vi "GetLastTotalGames.vi"(8 "error in (no error)":errorcluster, 11 "ClashRoyale in":refnum<class "ClashRoyale.lvclass">) -> (0 "error out":errorcluster, 2 "Last Total Games":i64, 3 "ClashRoyale out":refnum<class "ClashRoyale.lvclass">)   [LabVIEW 2020, in "ClashRoyale.lvclass"]
uses:
  ClashRoyale.lvclass
  <vilib>/drjdpowell/SQLite Library/SQLite.lvlib
  <vilib>/drjdpowell/SQLite Library/SQL Connection/Execute SQL (Single Integer).vi
  <vilib>/drjdpowell/SQLite Library/SQL Connection/Connection.lvclass
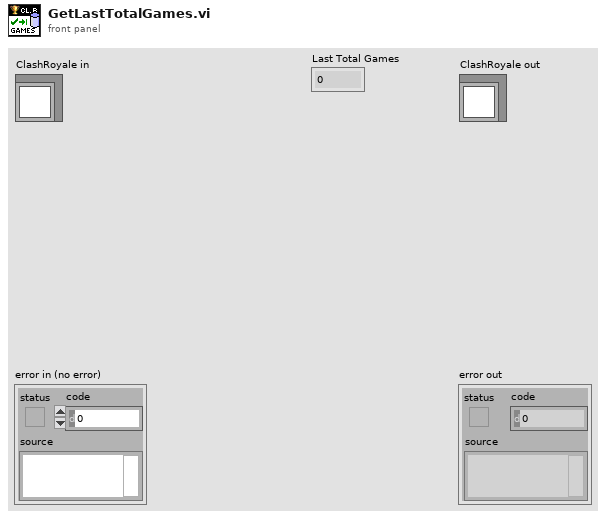
[diagram p1: front panel]
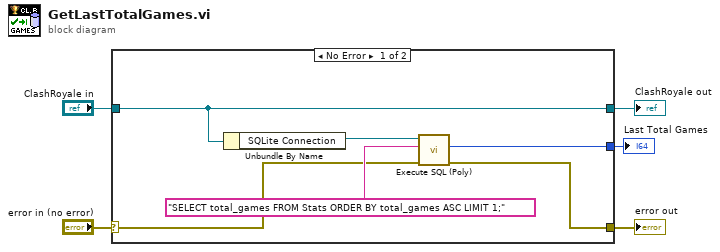
[diagram p0: block diagram]
diagram:
  n1 = case shown="No Error" "error in (no error)" {
    selector: "error in (no error)" -> [w7 w13]
    tunnel: [w6 w13] -> w4
    tunnel: [w11 w12] -> w2
    tunnel: "ClashRoyale in" -> [w11 w12]
    tunnel: [w8 _] -> w1
    frame No Error {
      n2 = Unbundle By Name(w11) -> ("SQLite Connection"=w10:refnum<class "Connection.lvclass">)
      n3 = call-poly <vilib>:"Execute SQL (Poly).vi"("error in (no error)"=w7, "SQL"="SELECT total_games FROM Stats ORDER BY total_games ASC LIMIT 1;", "SQLite Connection in"=w10) -> ("error out"=w6:errorcluster, "Result"=w8:i64)  [unwired: 6 in, 1 out]
    }
    frame Error {
    }
  }
  "error out" <- w4
  "ClashRoyale out" <- w2
  "Last Total Games" <- w1
